vi "Interface Error Info.vi"(11 "error":T1) -> (3 "error info":cluster{"code":i32, "description":string})   [LabVIEW 2017, in "DSF Core.lvlib" / "Interface.lvclass"]
uses:
  Interface.lvclass
  Errors.ctl
  Framework/Base Error Code.vi
  Framework/Framework.lvclass
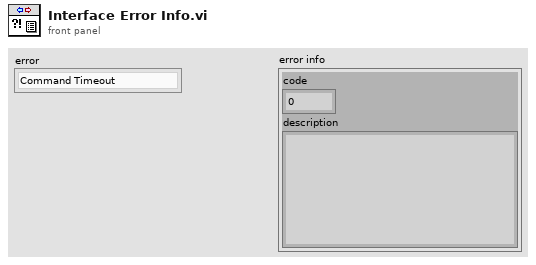
[diagram p1: front panel]
types:
  T1 = typedef "DSF Core.lvlib/Interface.lvclass/Errors.ctl" = enum16{"Command Timeout", "Response Timeout", "Error Timeout", "Invalid Response", "Invalid Response Parameters"}
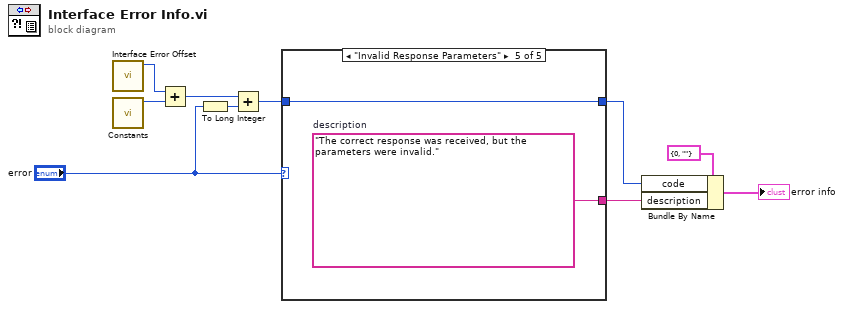
[diagram p0: block diagram]
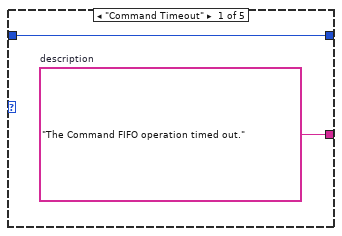
[diagram p2: hidden frame]
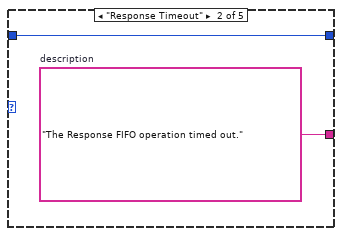
[diagram p3: hidden frame]
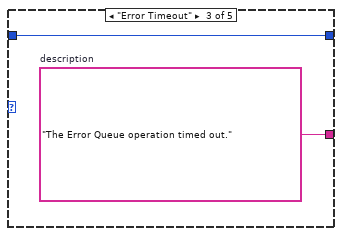
[diagram p4: hidden frame]
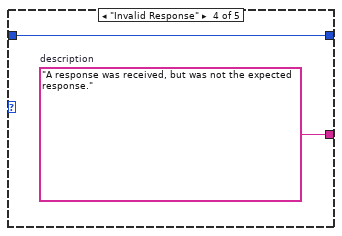
[diagram p5: hidden frame]
diagram:
  n1 = call "Interface Error Offset.vi"() -> ("base error offset"=w2:i32)  [unwired: 11 in]
  n2 = call-poly "Constants.vi"() -> ("base error code"=w10:i32)  [unwired: 11 in]
  n3 = Add(x=w2, y=w10) -> (x+y=w6:i32)
  n4 = To Long Integer(number="error") -> (32bit integer=w9:i32)
  n5 = Add(x=w6, y=w9) -> (x+y=w5:i32)
  n6 = case shown="\"Invalid Response Parameters\"" "error" {
    tunnel: [w12 w14 w16 w18 w20] -> w7
    tunnel: w5 -> [w11 w13 w15 w17 w19]
    tunnel: [w11 w13 w15 w17 w19] -> w4
    frame "Command Timeout" {
      w12 = "The Command FIFO operation timed out."  # description
    }
    frame "Response Timeout" {
      w14 = "The Response FIFO operation timed out."  # description
    }
    frame "Error Timeout" {
      w16 = "The Error Queue operation timed out."  # description
    }
    frame "Invalid Response" {
      w18 = "A response was received, but was not the expected response."  # description
    }
    frame "Invalid Response Parameters" {
      w20 = "The correct response was received, but the parameters were invalid."  # description
    }
  }
  n7 = Bundle By Name(cluster=cluster{"code":i32, "description":string} {"code"=0, "description"=""}, "code"=w4, "description"=w7) -> (→"error info":cluster{"code":i32, "description":string})
